vi "Logger Log Motor.vi"(6 "Log Quantity":enum16{"Verbose", "Sub1", "Sub2", "Minimal"}(ring), 7 "Precision Level (3)":i16=3, 8 "error in (no error)":errorcluster, 9 "Log Type":enum16{"Debug", "Info", "Error", "Warn"}(ring)=enum."Info", 10 "Motor Name":string, 11 "LoggerRef Name":string) -> (0 "error out":errorcluster)   [LabVIEW 2014]
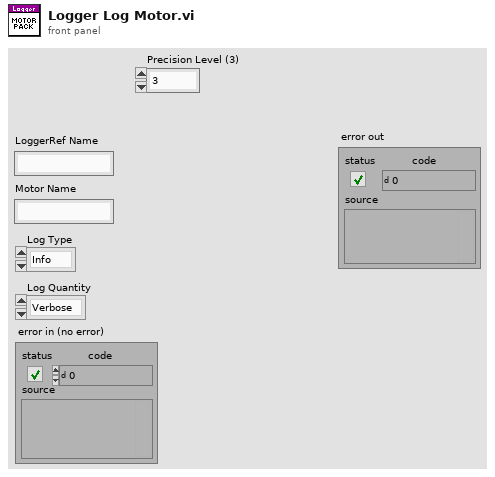
[diagram p1: front panel]
types:
  T1 = typedef "WPI_MotorControlDeviceRef.ctl" = cluster{"DeviceStatus":errorcluster, "Type":T2, "PWM":cluster{"Controller":T3, "PWM Channel":T4, "DeadBand":T5}, "CAN":cluster{"Device Number":u8, "Control Mode":T6, "Semaphore":T7, "Max Vout":dbl, "TalonSRX Control Mode":T8}, "Invert":bool, "TransformRef":T9, "InvTransformRef":T9}
  T2 = typedef "WPI_MotorControlType.ctl" = enum16{"PWM", "CAN", "CANTalonSRX"}
  T3 = typedef "FPGA_TypedefDigitalModule.ctl" = enum16{"Controller 1"}
  T4 = typedef "FPGA_DIOPWMChannel.ctl" = enum8{"PWM 0", "PWM 1", "PWM 2", "PWM 3", "PWM 4", "PWM 5", "PWM 6", "PWM 7", "PWM 8", "PWM 9", "PWM MXP 0", "PWM MXP 1", "PWM MXP 2", "PWM MXP 3", "PWM MXP 4", "PWM MXP 5", "PWM MXP 6", "PWM MXP 7", "PWM MXP 8", "PWM MXP 9", "Invalid"}
  T5 = typedef "WPI_PWMDeadband.ctl" = cluster{"Name":string, "maxPositivePwm":i32, "minPositivePwm":i32, "centerPwm":i32, "maxNegativePwm":i32, "minNegativePwm":i32, "angularRange":u16}
  T6 = typedef "WPI_CANJaguar_ControlMode.ctl" = enum8{"Percent VBus", "Current", "Speed", "Position", "Voltage"}
  T7 = typedef "Semaphore RefNum" = refnum<k1>
  T8 = typedef "WPI_CANTalonSRX_APIControlMode.ctl" = enum8{"Percent VBus", "Speed", "Position", "Slave", "Unchanged / Invalid"}
  T9 = typedef "WPI_PWMTransform_ConPane.ctl" = refnum<vi>
  T10 = typedef "LoggerRef.ctl" = cluster{"queueName":string, "queue":refnum<queue>, "queueError":errorcluster}
  T11 = typedef "WPI_CANTalonSRX_GlobalStatus.ctl" = cluster{"Applied Throttle":dbl, "Module Enabled":bool, "CAN Error":errorcluster, "Closed Loop Error":dbl, "Forward Limit Switch Closed":bool, "Reverse Limit Switch Closed":bool, "Sensor Position":dbl, "Sensor Velocity":dbl, "Current":dbl, "Sticky Fault - Over Temp":bool, "Sticky Fault - Under Voltage":bool, "Sticky Fault - Forward Limit":bool, "Sticky Fault - Reverse Limit":bool, "Sticky Fault - Forward Soft Limit":bool, "Sticky Fault - Reverse Soft Limit":bool, "Brake is Enabled":bool, "Encoder Position":dbl, "Encoder Velocity":dbl, "Encoder Index Count":dbl, "Encoder A Pin State":bool, "Encoder B Pin State":bool, "Encoder Index Pin State":bool, "Analog In":dbl, "Analog In Velocity":dbl, "Temperature (C)":dbl, "Battery Voltage":dbl}
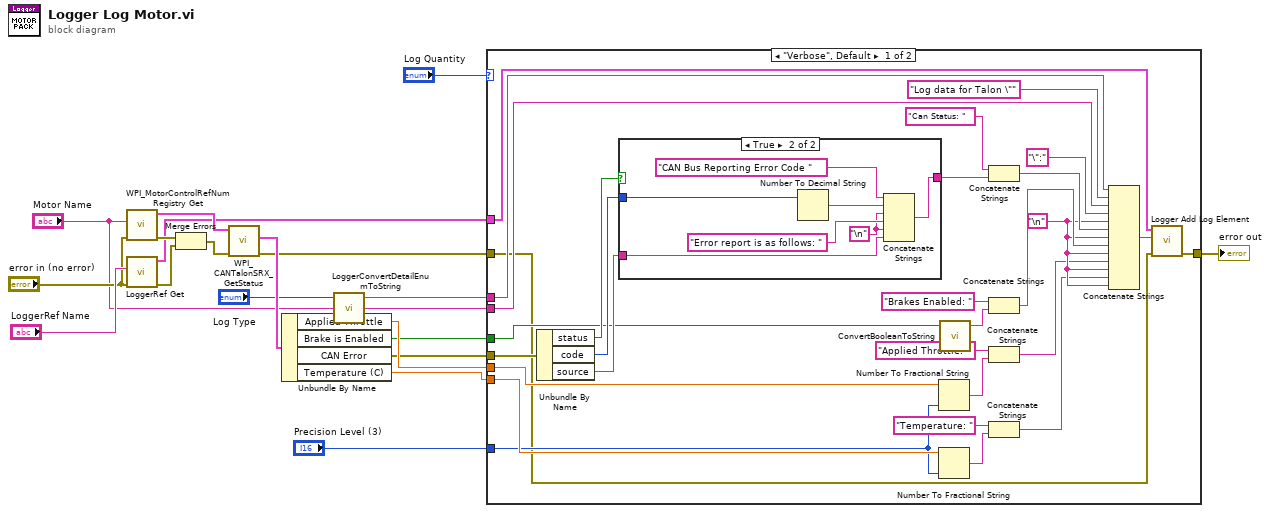
[diagram p0: block diagram]
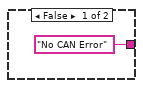
[diagram p2: hidden frame]
diagram:
  n1 = call <vilib>:"WPI_MotorControlRefNum Registry Get.vi"("error in (no error)"="error in (no error)", "refnum name"="Motor Name") -> ("error out"=w11:errorcluster, "MotorControlDevRef"=w14:T1)  [unwired: 8 in]
  n2 = call "LoggerRef Get.vi"("error in (no error)"="error in (no error)", "LoggerRef Name"="LoggerRef Name") -> ("error out"=w13:errorcluster, "LoggerRef Out"=w4:T10)  [unwired: 8 in]
  n3 = Merge Errors(w11, w13) -> (w12:errorcluster)
  n4 = call <vilib>:"WPI_CANTalonSRX_GetStatus.vi"("error in (no error)"=w12, "CAN Talon SRX Ref"=w14) -> ("error out"=w5:errorcluster, "Talon SRX Status"=w18:T11)  [unwired: 7 in, 1 out]
  n5 = Unbundle By Name(w18) -> ("Applied Throttle"=w17:dbl, "Brake is Enabled"=w2:bool, "CAN Error"=w10:errorcluster, "Temperature (C)"=w1:dbl)
  n6 = call "LoggerConvertDetailEnumToString.vi"("Log Type"="Log Type") -> ("String"=w8:string)  [unwired: 4 in]
  n7 = case shown="\"Verbose\", Default" "Log Quantity" {
    tunnel: w17 -> [w48 _]
    tunnel: w1 -> [w43 _]
    tunnel: w2 -> [w41 _]
    tunnel: w10 -> [w47 _]
    tunnel: w8 -> [w37 _]
    tunnel: "Precision Level (3)" -> [w42 _]
    tunnel: "Motor Name" -> [w38 _]
    tunnel: w5 -> [w21 w57]
    tunnel: w4 -> [w22 _]
    tunnel: [w20 w57] -> w3
    frame "Verbose", Default {
      w30 = "\n"
      n8 = Unbundle By Name(w47) -> ("status"=w46:bool, "code"=w45:i32, "source"=w44:string)
      n9 = case shown="True" w46 {
        tunnel: w45 -> [_ w56]
        tunnel: w44 -> [_ w51]
        tunnel: ["No CAN Error" w50] -> w39
        frame False {
        }
        frame True {
          w52 = "\n"
          n10 = Number To Decimal String(number=w56) -> (decimal integer string=w54:string)  [unwired: 1 in]
          n11 = Concatenate Strings("CAN Bus Reporting Error Code ", w54, w52, "Error report is as follows: " ("string"), w52, w51) -> (w50:string)
        }
      }
      n12 = Number To Fractional String(number=w48, precision (6)=w42) -> (F-format string=w25:string)  [unwired: 2 in]
      n13 = Number To Fractional String(number=w43, precision (6)=w42) -> (F-format string=w29:string)  [unwired: 2 in]
      n14 = call "ConvertBooleanToString.vi"("Boolean"=w41) -> ("String"=w33:string)  [unwired: 4 in]
      n15 = Concatenate Strings("Can Status: ", w39) -> (w34:string)
      n16 = Concatenate Strings("Brakes Enabled: " ("string"), w33) -> (w31:string)
      n17 = Concatenate Strings("Applied Throttle: ", w25) -> (w24:string)
      n18 = Concatenate Strings("Temperature: ", w29) -> (w27:string)
      n19 = Concatenate Strings(w37, "Log data for Talon \"" ("string"), w38, "\":" ("string"), w30, w34, w30, w31, w30, w24, w30, w27, w30) -> (w23:string)
      n20 = call "Logger Add Log Element.vi"("error in (no error)"=w21, "Element"=w23, "LoggerRef In"=w22) -> ("error out"=w20:errorcluster)  [unwired: 7 in, 1 out]
    }
    frame "Sub1" {
    }
  }
  "error out" <- w3
